vi "determineFilePaths.vi"(8 "error in (no error)":errorcluster, 11 "Logger in":refnum<class "Log.lvclass">) -> (0 "error out":errorcluster, 3 "Logger out":refnum<class "Log.lvclass">)   [LabVIEW 2013, in "Log.lvclass"]
uses:
  Log.lvclass
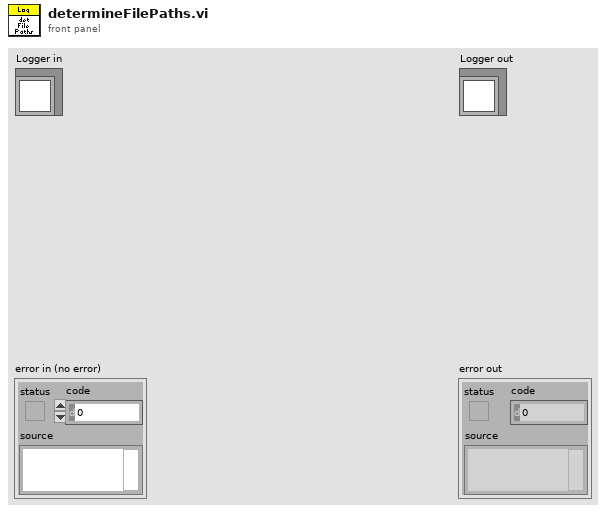
[diagram p1: front panel]
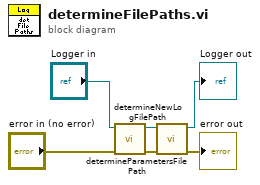
[diagram p0: block diagram]
diagram:
  n1 = call "determineNewLogFilePath.vi"("error in (no error)"="error in (no error)", "Logger in"="Logger in") -> ("error out"=w3:errorcluster, "Logger out"=w6:refnum<class "Log.lvclass">)  [unwired: 7 in, 1 out]
  n2 = call "determineParametersFilePath.vi"("error in (no error)"=w3, "Logger in"=w6) -> ("error out"=→"error out":errorcluster, "Logger out"=→"Logger out":refnum<class "Log.lvclass">)  [unwired: 8 in]
